vi "lockin - Set all f same.vi"(9 "all  frequencies same?":bool, 10 "Lockin":T1={"REF f (Hz)"=[13.0, 13.0, 13.0, 13.0, 13.0, 13.0, 13.0, 13.0], "REF phi (deg)"=[0.0, 0.0, 0.0, 0.0, 0.0, 0.0, 0.0, 0.0]} {"REF phi (deg)" format="%#_3g"}, 11 "AO":T2={"AO amp (V)"=[0.1, 0.09, 0.08, 0.07, 0.06, 0.05, 0.04, 0.03], "AO DC (V)"=[0.0, 0.0, 0.0, 0.0, 0.0, 0.0, 0.0, 0.0], "AO f (Hz)"=[13.0, 13.0, 13.0, 13.0, 13.0, 13.0, 13.0, 13.0], "AO phi (deg)"=[0.0, 0.0, 0.0, 0.0, 0.0, 0.0, 0.0, 0.0], "function"=[enum."Sine Wave", enum."Sine Wave", enum."Sine Wave", enum."Sine Wave", enum."Sine Wave", enum."Sine Wave", enum."Sine Wave", enum."Sine Wave"]} {"AO DC (V)" format="%#_6p"; "AO amp (V)" format="%#_6p"}) -> (2 "Lockin 2":T1={"REF f (Hz)"=[13.0, 13.0, 13.0, 13.0, 13.0, 13.0, 13.0, 13.0], "REF phi (deg)"=[0.0, 0.0, 0.0, 0.0, 0.0, 0.0, 0.0, 0.0]} {"REF phi (deg)" format="%#_3g"}, 3 "AO 2":T2={"AO amp (V)"=[0.1, 0.09, 0.08, 0.07, 0.06, 0.05, 0.04, 0.03], "AO DC (V)"=[0.0, 0.0, 0.0, 0.0, 0.0, 0.0, 0.0, 0.0], "AO f (Hz)"=[13.0, 13.0, 13.0, 13.0, 13.0, 13.0, 13.0, 13.0], "AO phi (deg)"=[0.0, 0.0, 0.0, 0.0, 0.0, 0.0, 0.0, 0.0], "function"=[enum."Sine Wave", enum."Sine Wave", enum."Sine Wave", enum."Sine Wave", enum."Sine Wave", enum."Sine Wave", enum."Sine Wave", enum."Sine Wave"]} {"AO DC (V)" format="%#_6p"; "AO amp (V)" format="%#_6p"})   [LabVIEW 2013]
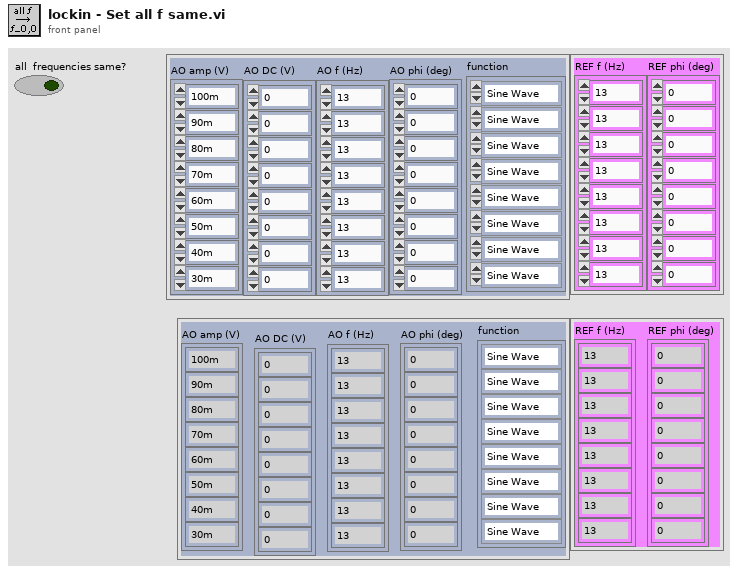
[diagram p1: front panel]
types:
  T1 = cluster{"REF f (Hz)":dbl[], "REF phi (deg)":dbl[]}
  T2 = cluster{"AO amp (V)":dbl[], "AO DC (V)":dbl[], "AO f (Hz)":dbl[], "AO phi (deg)":dbl[], "function":enum16{"Sine Wave", "Triangle Wave", "Square Wave", "Sawtooth Wave"}[]}
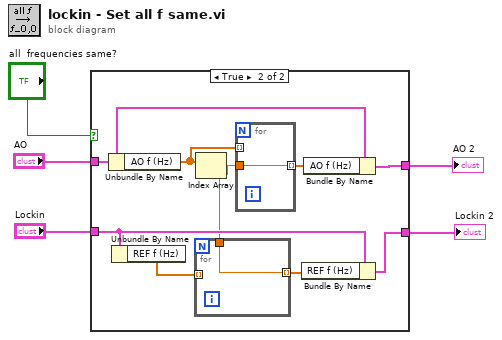
[diagram p0: block diagram]
diagram:
  n1 = case shown="True" "all  frequencies same?" {
    tunnel: "AO" -> [w7 w16]
    tunnel: [w7 w15] -> w3
    tunnel: "Lockin" -> [w6 w12]
    tunnel: [w6 w14] -> w2
    frame False {
    }
    frame True {
      n2 = Unbundle By Name(w16) -> ("AO f (Hz)"=w8:dbl[])
      n3 = Unbundle By Name(w12) -> ("REF f (Hz)"=w13:dbl[])
      n4 = Index Array(array=w8) -> (element=w10:dbl)  [unwired: 1 in]
      n5 = for {
        tunnel: w13 -> [_] mode=indexing
        tunnel: [w18] -> w11 mode=indexing
        tunnel: w10 -> [w18]
      }
      n6 = for {
        tunnel: w10 -> [w17]
        tunnel: [w17] -> w9 mode=indexing
        tunnel: w8 -> [_] mode=indexing
      }
      n7 = Bundle By Name(cluster=w12, "REF f (Hz)"=w11) -> (w14:T1)
      n8 = Bundle By Name(cluster=w16, "AO f (Hz)"=w9) -> (w15:T2)
    }
  }
  "AO 2" <- w3
  "Lockin 2" <- w2
